vi "round number to decimal.vi"(9 "y":dbl, 10 "x":dbl) -> (2 "rounded number":dbl)   [LabVIEW 2019]
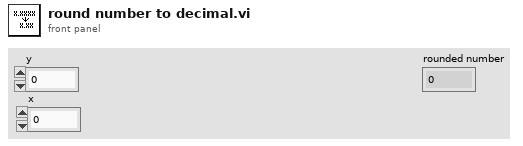
[diagram p1: front panel]
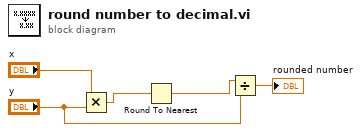
[diagram p0: block diagram]
diagram:
  n1 = Multiply(x="x", y="y") -> (x*y=w5:dbl)
  n2 = Round To Nearest(number=w5) -> (nearest integer value=w2:dbl)
  n3 = Divide(x=w2, y="y") -> (x/y=→"rounded number":dbl)
